vi "Test Deserialize Variants.vi"(8 "error in (no error)":errorcluster) -> (0 "error out":errorcluster)   [LabVIEW 2013]
uses:
  src/Deserializer/JSON Deserializer/JSON Deserializer.lvclass
  <vilib>/addons/_JKI Toolkits/Caraya/classes/Test/Test.lvclass
  <vilib>/addons/_JKI Toolkits/Caraya/classes/Assert/Assert.lvclass
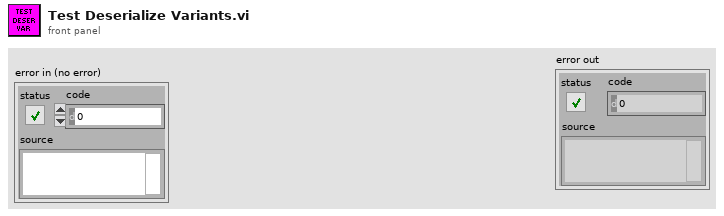
[diagram p1: front panel]
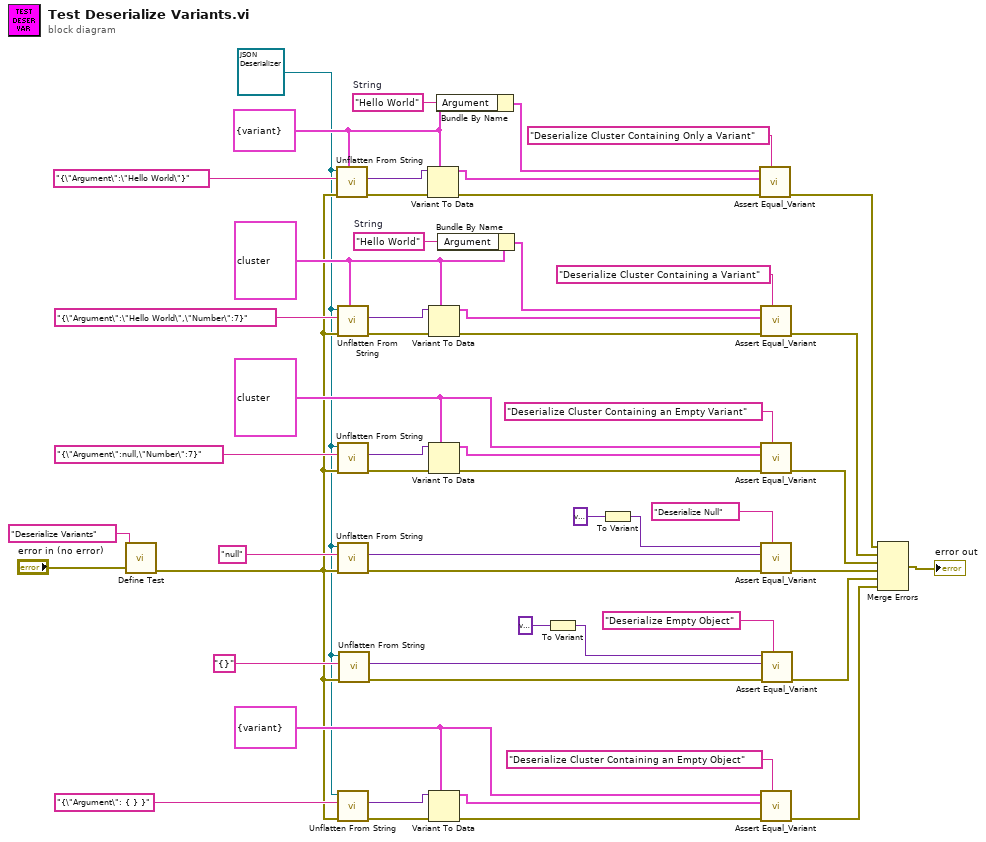
[diagram p0: block diagram]
diagram:
  w4 = cluster{"Argument":variant} {"Argument"=variant}
  w20 = cluster{"Argument":variant, "Number":i32} {"Argument"=variant, "Number"=7}
  w31 = "Hello World"  # String
  w34 = cluster{"Argument":variant} {"Argument"=variant}
  w44 = "Hello World"  # String
  w41 = cluster{"Argument":variant, "Number":i32} {"Argument"=variant, "Number"=7}
  w2 = refnum<class "JSON Deserializer.lvclass"> refnum ("Deserializer out")
  n1 = call <vilib>:"Define Test.vi"("error in (no error)"="error in (no error)", "Label (VI Title)"="Deserialize Variants") -> ("error out"=w3:errorcluster)  [unwired: 9 in]
  n2 = call-dynamic "Unflatten From String.vi"("Type and Defaults"=w34, "error in (no error)"=w3, "String"="{\"Argument\":\"Hello World\"}", "Deserializer in"=w2) -> ("error out"=w33:errorcluster, "Variant"=w32:variant)  [unwired: 5 in, 1 out]
  n3 = call-dynamic "Unflatten From String.vi"("Type and Defaults"=w41, "error in (no error)"=w3, "String"="{\"Argument\":\"Hello World\",\"Number\":7}", "Deserializer in"=w2) -> ("error out"=w42:errorcluster, "Variant"=w43:variant)  [unwired: 5 in, 1 out]
  n4 = call-dynamic "Unflatten From String.vi"("error in (no error)"=w3, "String"="{\"Argument\":null,\"Number\":7}", "Deserializer in"=w2) -> ("error out"=w25:errorcluster, "Variant"=w24:variant)  [unwired: 6 in, 1 out]
  n5 = call-dynamic "Unflatten From String.vi"("error in (no error)"=w3, "String"="null", "Deserializer in"=w2) -> ("error out"=w49:errorcluster, "Variant"=w48:variant)  [unwired: 6 in, 1 out]
  n6 = call-dynamic "Unflatten From String.vi"("error in (no error)"=w3, "String"="{\"Argument\": { } }", "Deserializer in"=w2) -> ("error out"=w8:errorcluster, "Variant"=w7:variant)  [unwired: 6 in, 1 out]
  n7 = call-dynamic "Unflatten From String.vi"("error in (no error)"=w3, "String"="{}", "Deserializer in"=w2) -> ("error out"=w15:errorcluster, "Variant"=w14:variant)  [unwired: 6 in, 1 out]
  n8 = Variant To Data(error in=w33, type=w34, Variant=w32) -> (data=w35:cluster{"Argument":variant}, error out=w37:errorcluster)
  n9 = Variant To Data(error in=w42, type=w41, Variant=w43) -> (data=w40:cluster{"Argument":variant, "Number":i32}, error out=w38:errorcluster)
  n10 = Variant To Data(error in=w25, type=w20, Variant=w24) -> (data=w26:cluster{"Argument":variant, "Number":i32}, error out=w27:errorcluster)
  n11 = Variant To Data(error in=w8, type=w4, Variant=w7) -> (data=w9:cluster{"Argument":variant}, error out=w10:errorcluster)
  n12 = Bundle By Name(cluster=w34, "Argument"=w31) -> (w36:cluster{"Argument":variant})
  n13 = Bundle By Name(cluster=w41, "Argument"=w44) -> (w39:cluster{"Argument":variant, "Number":i32})
  n14 = To Variant(anything=variant ("Variant")) -> (Variant=w12:variant)
  n15 = To Variant(anything=variant ("Variant")) -> (Variant=w18:variant)
  n16 = call <vilib>:"Assert Equal_Variant.vi"("Label"="Deserialize Cluster Containing Only a Variant", "error in (no error)"=w37, "Y"=w35, "X"=w36) -> ("error out"=w28:errorcluster)  [unwired: 7 in]
  n17 = call <vilib>:"Assert Equal_Variant.vi"("Label"="Deserialize Cluster Containing a Variant", "error in (no error)"=w38, "Y"=w40, "X"=w39) -> ("error out"=w46:errorcluster)  [unwired: 7 in]
  n18 = call <vilib>:"Assert Equal_Variant.vi"("Label"="Deserialize Cluster Containing an Empty Variant", "error in (no error)"=w27, "Y"=w26, "X"=w20) -> ("error out"=w21:errorcluster)  [unwired: 7 in]
  n19 = call <vilib>:"Assert Equal_Variant.vi"("Label"="Deserialize Null", "error in (no error)"=w49, "Y"=w48, "X"=w18) -> ("error out"=w52:errorcluster)  [unwired: 7 in]
  n20 = call <vilib>:"Assert Equal_Variant.vi"("Label"="Deserialize Cluster Containing an Empty Object", "error in (no error)"=w10, "Y"=w9, "X"=w4) -> ("error out"=w1:errorcluster)  [unwired: 7 in]
  n21 = call <vilib>:"Assert Equal_Variant.vi"("Label"="Deserialize Empty Object", "error in (no error)"=w15, "Y"=w14, "X"=w12) -> ("error out"=w11:errorcluster)  [unwired: 7 in]
  n22 = Merge Errors(w28, w46, w21, w52, w11, w1) -> (→"error out":errorcluster)
